vi "Run Data Acquisition.vi"(5 "output cluster 2":T2, 6 "Thresholding Cluster 2":T1={"F_DEx"=0, "F_AA"=0, " No of Bins"=100}, 8 "error in (no error)":errorcluster, 9 "Time Limit":dbl=1.0, 10 "Save Data":bool=TRUE, 11 "refnum in":refnum<file>) -> (0 "error out":errorcluster, 3 "refnum out":refnum<file>)   [LabVIEW 2009]
uses:
  Acquisition Settings.vi
panel:
  in  "Delta delay OFF-ON,ns":u32=3000
  in  "Delay ON,ns":u32=6000
  out "Number of Photons Counted":i32
  out "Arrival Time Clusters":T3(array[cluster])
  out "Update Time Out":dbl=28.253000000011546 format="%.2f"
  out "Timer Value (s)":dbl=28.25534135 format="%.2f"
  in  "stop":bool
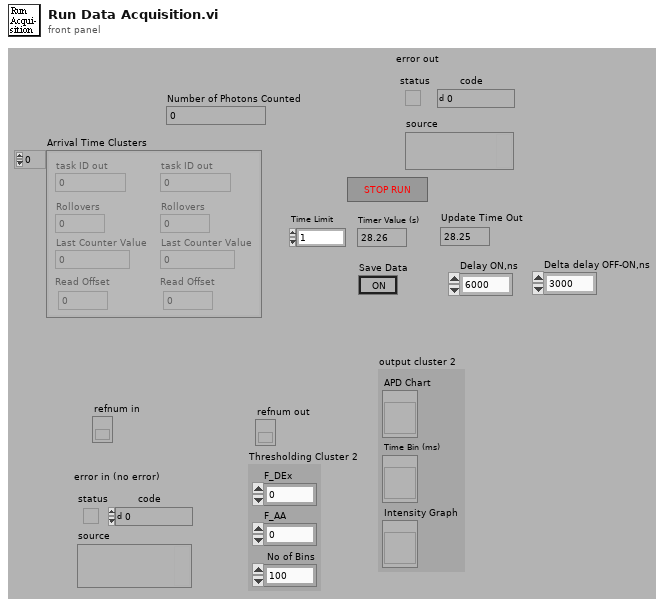
[diagram p1: front panel]
types:
  T1 = cluster{"F_DEx":i32, "F_AA":i32, " No of Bins":i32}
  T2 = cluster{"APD Chart":refnum<vi>, "Time Bin (ms)":refnum<vi>, "Intensity Graph":refnum<vi>}
  T3 = cluster{"task ID out":u32, "Rollovers":i32, "Last Counter Value":u32, "Read Offset":i32}[]
  T4 = cluster{"Name":string, "Device Number":i16, "Counter Number":i16, "Pulse Spec 1 (Clocks)":u32, "Pulse Spec 2 (Clocks)":u32, "Signal Routing Configuration":i16, "Inverted":bool}[]
  T5 = cluster{"Name":string, "Device Number":i16, "Counter Number":i16, "Pulse Spec 1 (Clocks)":u32, "Pulse Spec 2 (Clocks)":u32, "Signal Routing Configuration":i16, "Inverted":bool}
  T6 = cluster{string, "Resolution":dbl, "Offset":dbl, "Array Constant":string[]}[]
  T7 = cluster{"Type":string, "Byte Stream File Refnum":refnum<file>}
  T8 = cluster{"Last Counter Value":u32, "Rollovers":i32}
  T9 = cluster{"Type":string, "Byte Stream File Refnum":refnum<file>}[]
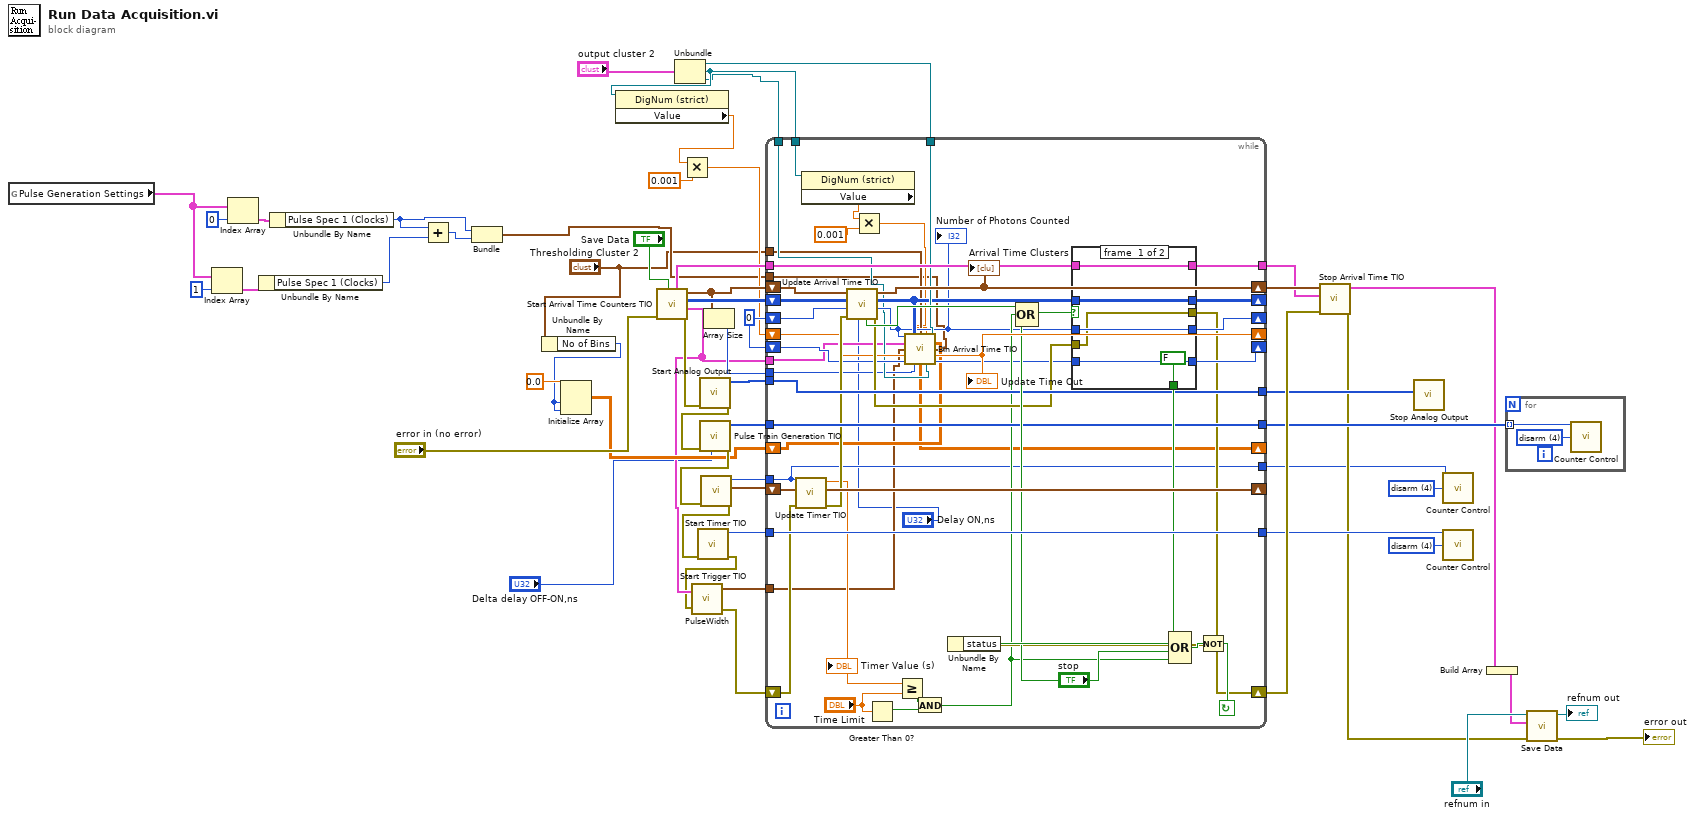
[diagram p0: block diagram]
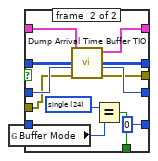
[diagram p2: hidden frame]
diagram:
  w21 = u32 4 items=["program", "reset", "arm", "prepare", "disarm", "count up", "count down", "switch cycle", "snapshot"] ("control code")
  w35 = 0
  w49 = u32 4 items=["program", "reset", "arm", "prepare", "disarm", "count up", "count down", "switch cycle", "snapshot"] ("control code")
  n1 = global read "Acquisition Settings.vi" "Pulse Generation Settings"() -> (w8:T4)
  n2 = Index Array(array=w8, index=1) -> (element=w9:T5)
  n3 = Index Array(array=w8, index=0) -> (element=w10:T5)
  n4 = Unbundle By Name(w9) -> ("Pulse Spec 1 (Clocks)"=w7:u32)
  n5 = Unbundle By Name(w10) -> ("Pulse Spec 1 (Clocks)"=w6:u32)
  n6 = Add(x=w6, y=w7) -> (x+y=w5:u32)
  n7 = Bundle("Pulse Spec 1 (Clocks)"=w6, w5) -> (w4:cluster{"Pulse Spec 1 (Clocks)":u32, u32})  [unwired: 1 in]
  n8 = Unbundle By Name("Thresholding Cluster 2") -> ("No of Bins"=w2:i32)
  n9 = Initialize Array(0.0 ("element"), w2, w2) -> (w17:dbl[][])
  n10 = call "Start Arrival Time Counters TIO.vi"("Save Data"="Save Data", "error in"="error in (no error)") -> ("error out"=w43:errorcluster, "Column Definitions"=w15:T6, "Buffer"=w34:i32[][], "Arrival Time Clusters"=w33:T3, "Temp File Definition"=w36:T7)  [unwired: 5 in]
  n11 = Unbundle("output cluster 2") -> ("APD Chart"=w26:refnum<vi>, "Time Bin (ms)"=w24:refnum<vi>, "Intensity Graph"=w20:refnum<vi>)
  n12 = property class="DigNum (strict)"(reference=w24) -> ("Value"=w25:dbl)  [unwired: 1 in, 2 out]
  n13 = Multiply(x=w25, y=0.001) -> (x*y=w27:dbl)
  n14 = call "Start Analog Output.vi"("error in (no error)"=w43) -> ("error out"=w40:errorcluster, "AO Task ID's Out"=w42:u32[])  [unwired: 9 in]
  n15 = call "Pulse Train Generation TIO.vi"("Delay"="Delta delay OFF-ON,ns", "error in"=w40) -> ("error out"=w41:errorcluster, "Pulse Generation Task ID's Out"=w39:u32[])  [unwired: 8 in]
  n16 = call "Start Timer TIO.vi"("error in"=w41) -> ("error out"=w53:errorcluster, "Timer Cluster Out"=w50:T8, "Timer task ID out"=w54:u32)  [unwired: 8 in]
  n17 = call "Start Trigger TIO.vi"("error in"=w53) -> ("error out"=w13:errorcluster, "Trigger task ID out"=w52:u32)  [unwired: 9 in]
  n18 = call "PulseWidth.vi"("Column Definitions 2"=w15, "error in"=w13) -> ("Pulse Width Cluster"=w16:cluster{dbl, dbl}, "error out"=w14:errorcluster)  [unwired: 1 in]
  n19 = Array Size(array=w33) -> (size(s)=w32:i32)
  n20 = while {
    tunnel: [w72] -> w22
    shift-left: w35 -> [w68]
    shift-right: [w86] -> _
    tunnel: [w87] -> w31
    tunnel: w32 -> [w64]
    tunnel: w15 -> [w58]
    tunnel: w36 -> [w90]
    tunnel: [w92] -> w38
    tunnel: [w93] -> w37
    tunnel: w39 -> [w92]
    tunnel: w42 -> [w93]
    tunnel: [w98] -> w48
    shift-left: w50 -> [w101]
    shift-right: [w100] -> _
    tunnel: w52 -> [w98]
    tunnel: w54 -> [w72]
    shift-left: w27 -> [w69]
    shift-right: [w103] -> _
    shift-left: w35 -> [w88]
    shift-right: [w102] -> _
    shift-left: w33 -> [w104]
    shift-right: [w91] -> w55
    shift-left: w34 -> [w105]
    shift-right: [w99] -> _
    shift-left: w14 -> [w81]
    shift-right: [w74] -> w51
    tunnel: w26 -> [w84]
    tunnel: w24 -> [w83]
    tunnel: w20 -> [w65]
    shift-right: [w63] -> _
    shift-left: w17 -> [w66]
    tunnel: "Thresholding Cluster 2" -> [w62]
    tunnel: w16 -> [w60]
    tunnel: w4 -> [w59]
    stop <- w106 continue-if-true
    n21 = call "Update Timer TIO.vi"("error in (no error)"=w81, "Timer Cluster"=w101, "task ID"=w72) -> ("error out"=w80:errorcluster, "Timer Cluster Out"=w100:T8, "Timer Value (s)"=w79:dbl)  [unwired: 6 in]
    "Timer Value (s)" <- w79
    n22 = property class="DigNum (strict)"(reference=w83) -> ("Value"=w82:dbl)  [unwired: 1 in, 2 out]
    n23 = call "Update Arrival Time TIO.vi"("Delay, ns"="Delay ON,ns", "error in"=w80, "Number of Photons Counted"=w88, "Buffer In"=w105, "Arrival Time Clusters"=w104) -> ("error out"=w75:errorcluster, "Number of Photons Counted Out"=w70:i32, "Buffer Out"=w71:i32[][], "Arrival Time Clusters"=w91:T3, "Dump Buffer"=w89:bool)  [unwired: 2 in]
    "Arrival Time Clusters" <- w91
    "Number of Photons Counted" <- w70
    n24 = Multiply(x=w82, y=0.001) -> (x*y=w61:dbl)
    n25 = Greater Than 0?(x="Time Limit") -> (x > 0?=w77:bool)
    n26 = Greater Or Equal?(x=w79, y="Time Limit") -> (x >= y?=w76:bool)
    n27 = call "Bin Arrival Time TIO.vi"("Read Position"=w70, "Array In"=w71, "Thresholding Cluster 2"=w62, "Time Bin (s)"=w61, "APD Chart 2"=w84, "Column Definitions"=w58, "Histogram In"=w66, "Pulse Width Cluster 2"=w60, "Pulse Widths"=w59, "Update Time In"=w69, "Binning Position"=w68, "Number of Channels"=w64, "Intensity Graph"=w65) -> ("Update Time Out"=w103:dbl, "Histogram Out"=w63:dbl[][], "Binning Position Out"=w67:i32)
    "Update Time Out" <- w103
    n28 = And(x=w76, y=w77) -> (x .and. y?=w73:bool)
    n29 = Compound Arithmetic op=OR(w89, w73, "stop") -> (w94:bool)
    n30 = case shown="True" w94 {
      tunnel: w70 -> [w113 w119]
      tunnel: [w113 w118] -> w102
      tunnel: [FALSE w122] -> w96
      tunnel: w71 -> [w111 w121]
      tunnel: [w111 w121] -> w99
      tunnel: w90 -> [w110 w120]
      tunnel: [w110 w117] -> w87
      tunnel: w67 -> [w109 _]
      tunnel: [w109 0 ("Binning Position Out")] -> w86
      tunnel: w75 -> [w108 w115]
      tunnel: [w108 w114] -> w74
      frame #0 {
      }
      frame #1 {
        w124 = u32 24 items=["yes", "no", "positive", "negative", "high", "low", "low to high", "high to low", "default", "max timebase", "other counter gate", "other counter TC", "other counter output", "other counter source", "source", "gate", "aux line", "in start trigger", "in stop trigger", "automatic", "enabled", "count up", "count down", "hardware", "single", "double", "pulse", "toggle", "quadrature encoder X1", "quadrature encoder X2", "quadrature encoder X4", "two pulse counting", "A high B high", "A high B low", "A low B high", "A low B low", "PFI n", "RTSI n", "timebase n"] ("Buffer Mode")
        n31 = global read "Acquisition Settings.vi" "Buffer Mode"() -> (w123:u32)
        n32 = call "Dump Arrival Time Buffer TIO.vi"("error in"=w115, "Number of Photons Counted"=w119, "Buffer In"=w121, "Temp File Definition"=w120) -> ("error out"=w114:errorcluster, "Number of Photons Counted Out"=w118:i32, "Temp File Definition Out"=w117:T7)  [unwired: 5 in]
        n33 = Equal?(x=w124, y=w123) -> (x = y?=w122:bool)
      }
    }
    n34 = Unbundle By Name(w74) -> ("status"=w97:bool)
    n35 = Compound Arithmetic op=OR(w96, w97, "stop", w73) -> (w107:bool)
    n36 = Not(x=w107) -> (.not. x?=w106:bool)
  }
  n37 = call "Stop Arrival Time TIO.vi"("error in"=w51, "Temp File Definition"=w31, "Arrival Time Clusters"=w55) -> ("error out"=w23:errorcluster, "Temp File Definition Out"=w30:T7)  [unwired: 7 in]
  n38 = call "Stop Analog Output.vi"("AO Task ID's In"=w37) -> ()  [unwired: 10 in, 1 out]
  n39 = call <vilib>:"Counter Control.vi"("task ID"=w22, "control code"=w21) -> ()  [unwired: 12 in, 2 out]
  n40 = call <vilib>:"Counter Control.vi"("task ID"=w48, "control code"=w49) -> ()  [unwired: 12 in, 2 out]
  n41 = Build Array(w30) -> (w29:T9)
  n42 = for {
    tunnel: w38 -> [w125] mode=indexing
    w126 = u32 4 items=["program", "reset", "arm", "prepare", "disarm", "count up", "count down", "switch cycle", "snapshot"] ("control code")
    n43 = call <vilib>:"Counter Control.vi"("task ID"=w125, "control code"=w126) -> ()  [unwired: 12 in, 2 out]
  }
  n44 = call "Save Data.vi"("error in (no error)"=w23, "Temp File Array"=w29, "refnum in"="refnum in") -> ("error out"=→"error out":errorcluster, "refnum out"=→"refnum out":refnum<file>)  [unwired: 6 in, 1 out]
